vi "PID_controller_04.vi"() -> ()   [LabVIEW 2011]
uses:
  <vilib>/Platform/TimedLoop/XDataNode/nitl_modes.ctl
  <vilib>/Platform/TimedLoop/XDataNode/timing_clust.ctl
  <vilib>/Platform/TimedLoop/XDataNode/wakeup.ctl
  <vilib>/Platform/TimedLoop/XDataNode/XDataNode.xnode
  <vilib>/Platform/TimedLoop/XDataNode/XDNodeRunTimeDep.lvlib
panel:
  out "prev value":dbl
  out "Numeric":dbl
  out "x-y":dbl
  out "S00":dbl
  out "S10":dbl
  out "S20":dbl
  out "S11":dbl
  out "S01":dbl
  out "weight":dbl[](array[numeric])
  in  "# of points to watch":i32
  in  "alpha":dbl=-1.0
  out "t0":dbl
  out "error(t)":cluster{dbl, "Value":dbl}[](array[cluster])
  out "error out":errorcluster
  out "first":bool=TRUE
  out "P (torr)":string
  out "XY Graph":T1(graph)
  out "current value":dbl
  in  "stop":bool
  in  "Period (s)":dbl
  out "dValue":dbl
  out "derivative":dbl
  out "integral":dbl
  out "error":dbl
  out "Current angle (deg)":dbl
  in  "Kd":dbl
  in  "Ki":dbl
  in  "Kp":dbl
  out "Current P (torr)":dbl
  in  "Set Point (torr)":dbl
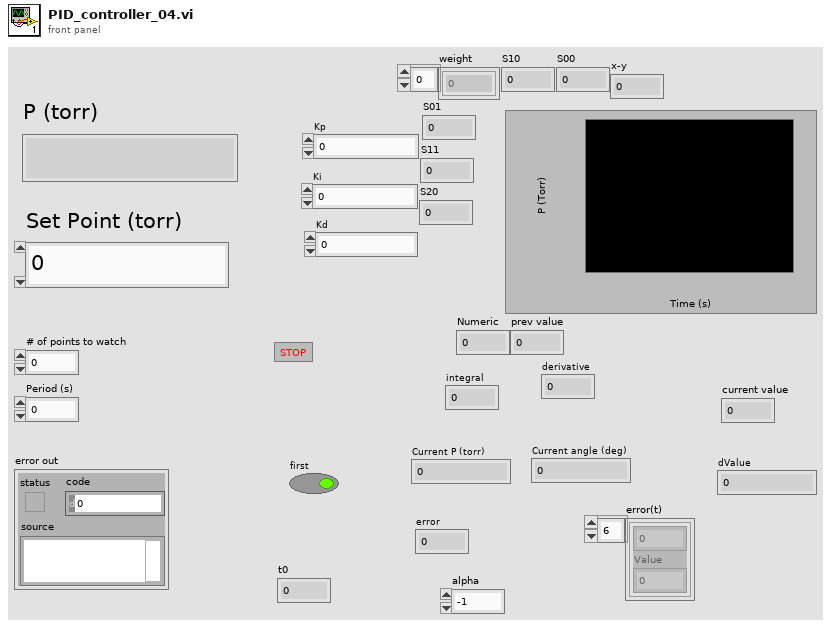
[diagram p1: front panel]
types:
  T1 = cluster{"Value":cluster{"element":dbl, "element":dbl}[]}[]
  T2 = typedef "XDNodeRunTimeDep.lvlib/nitl_modes.ctl" = enum32{"No Change", "Process missed periods, maintain original phase", "Discard missed periods, maintain original phase", "Process missed periods, ignore original phase", "Discard missed periods, ignore original phase"}
  T3 = typedef "XDNodeRunTimeDep.lvlib/timing_clust.ctl" = cluster{"Expected End [f-1]":u64, "Actual End [f-1]":u64, "Finished Late? [f-1]":bool, "Expected End [i-1]":u64, "Actual End [i-1]":u64, "Finished Late? [i-1]":bool, "Expected Start [i]":u64, "Actual Start [i]":u64, "Expected Start [f]":u64, "Actual Start [f]":u64, "Source Name":string, "Structure Name":string, "Period":i64, "Deadline":i64, "Offset":i64, "Start":i64, "Priority":i32, "Timeout":i32, "Mode":T2, "Wakeup Reason":T4, "Error":errorcluster, "Source Type":string, "Secondary Source Type":string, "Global End Time":u64, "Global Start Time":u64, "Frame Duration":u64, "Iteration Duration":u64, "Assigned CPU":i32, "I/O Scan Engine Mode":u32}
  T4 = typedef "XDNodeRunTimeDep.lvlib/wakeup.ctl" = enum32{"Normal", "Aborted", "Asynchronous wakeup", "Timing source error", "Timed loop error", "Timeout"}
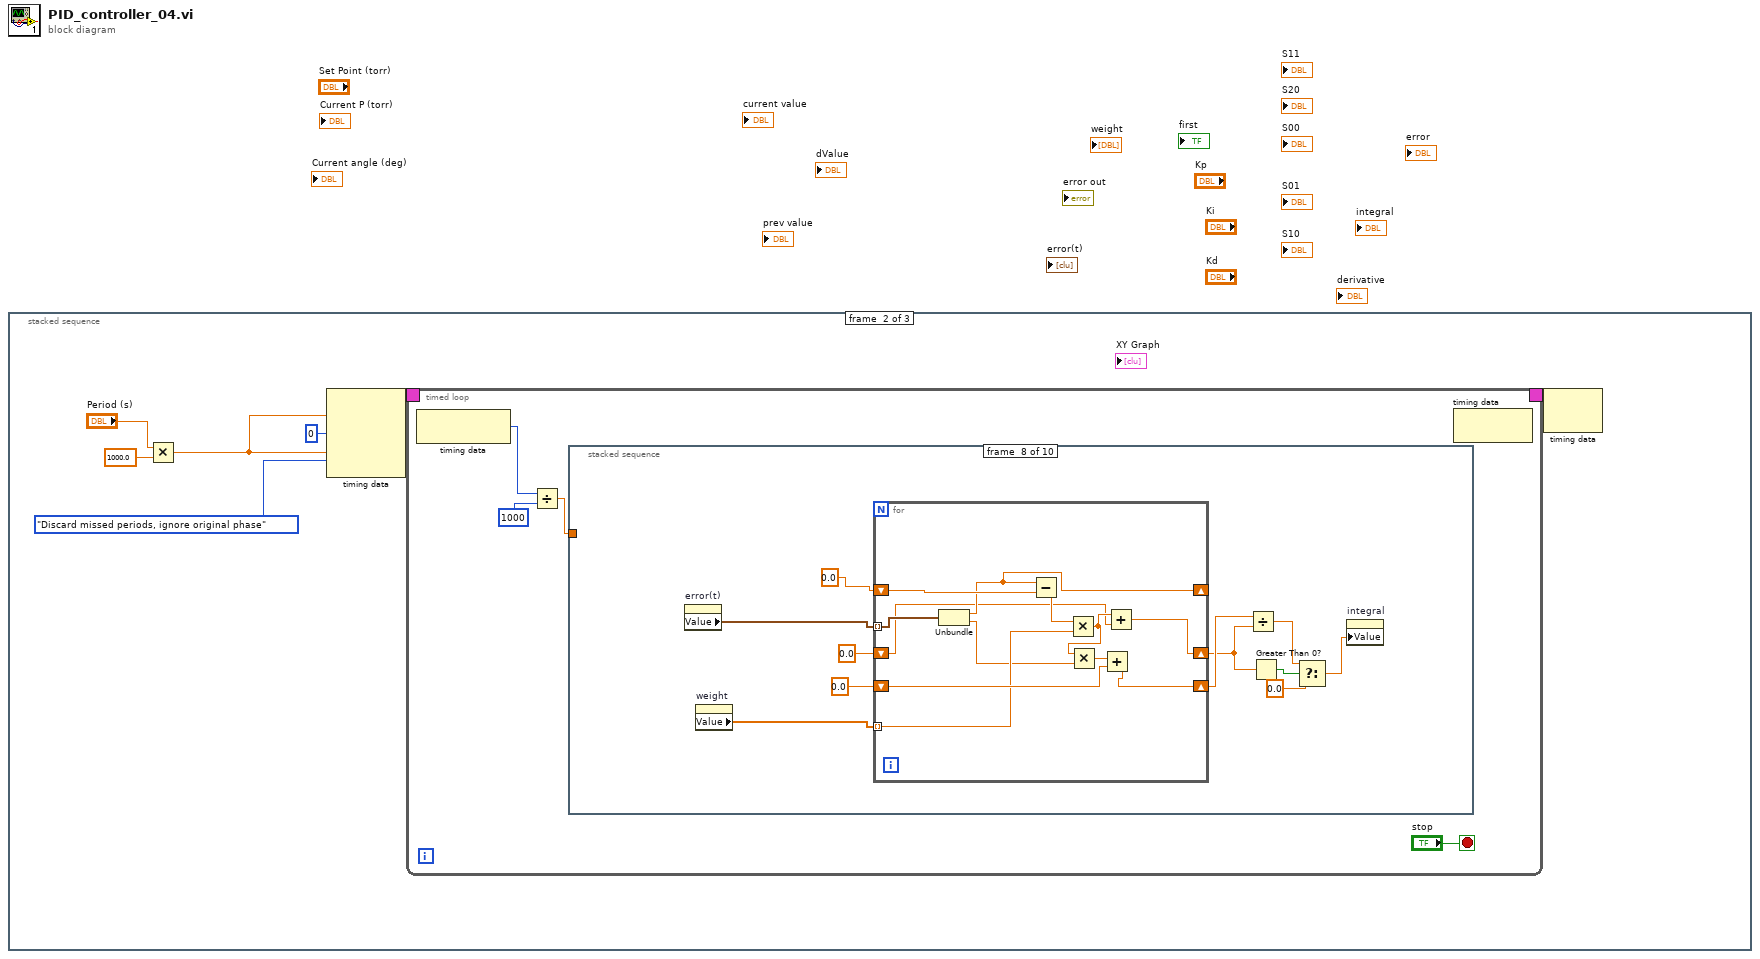
[diagram p0: block diagram]
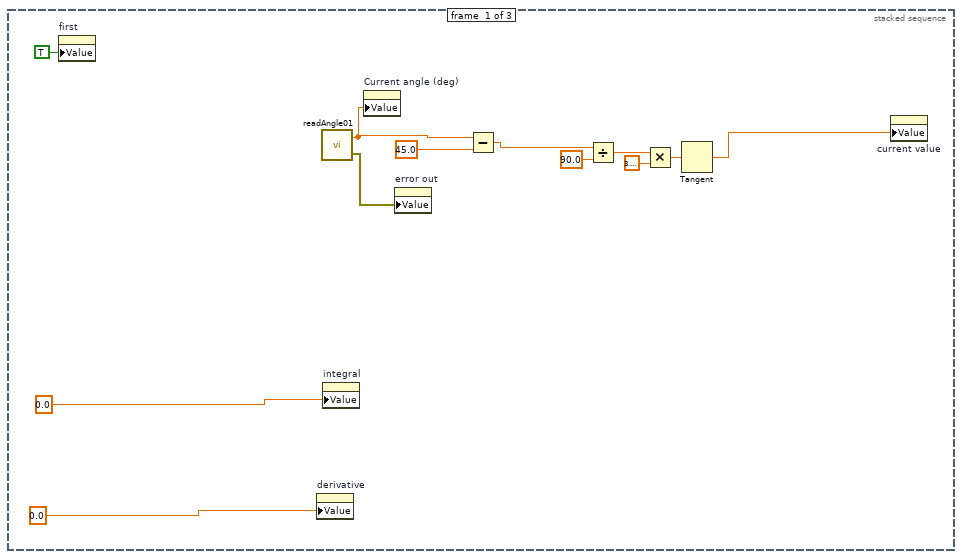
[diagram p2: hidden frame]
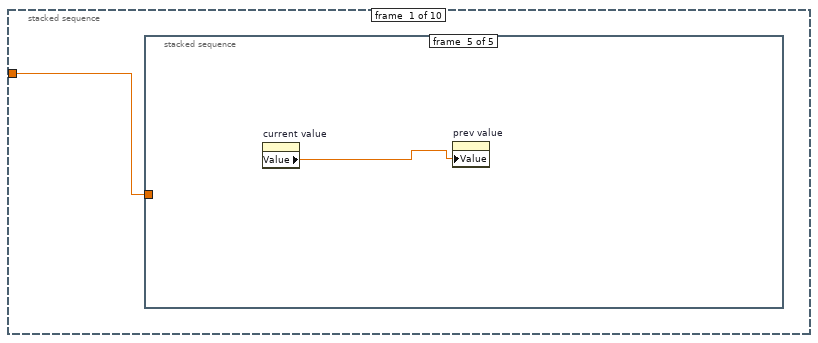
[diagram p3: hidden frame]
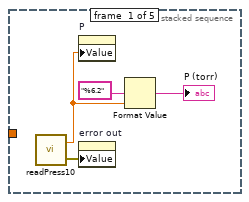
[diagram p4: hidden frame]
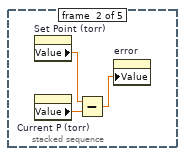
[diagram p5: hidden frame]
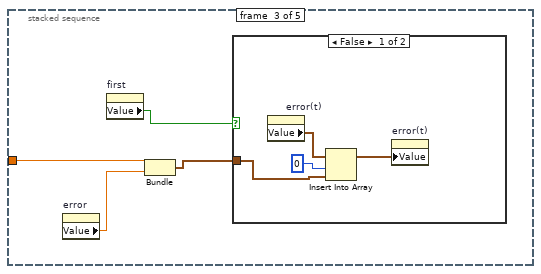
[diagram p6: hidden frame]
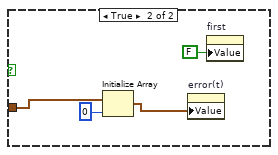
[diagram p7: hidden frame]
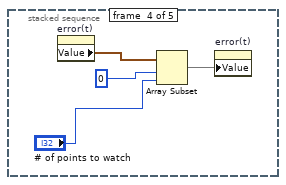
[diagram p8: hidden frame]
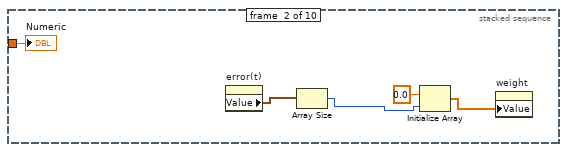
[diagram p9: hidden frame]
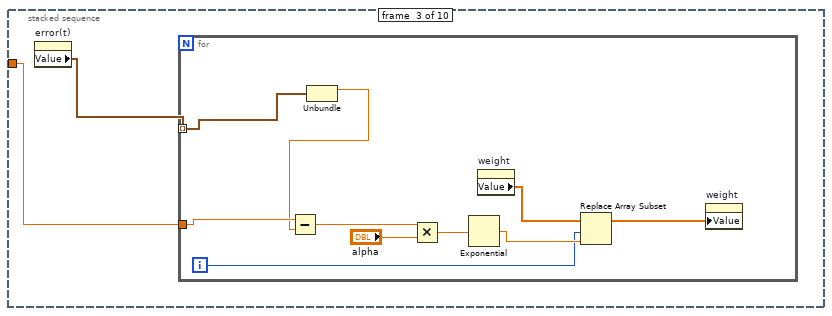
[diagram p10: hidden frame]
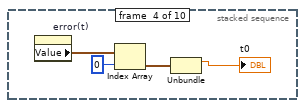
[diagram p11: hidden frame]
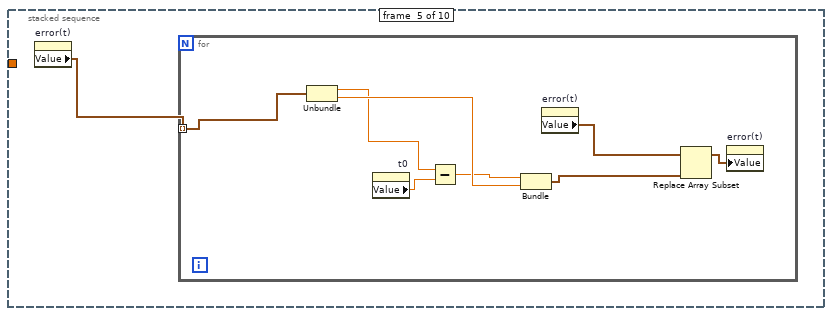
[diagram p12: hidden frame]
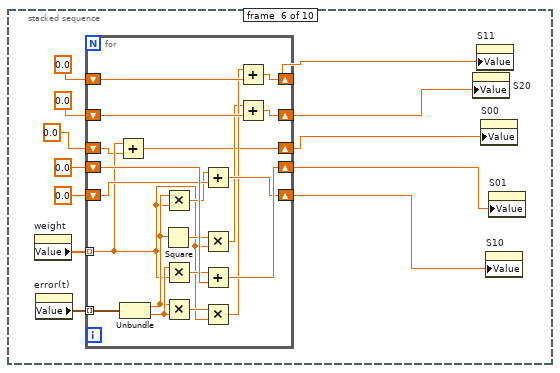
[diagram p13: hidden frame]
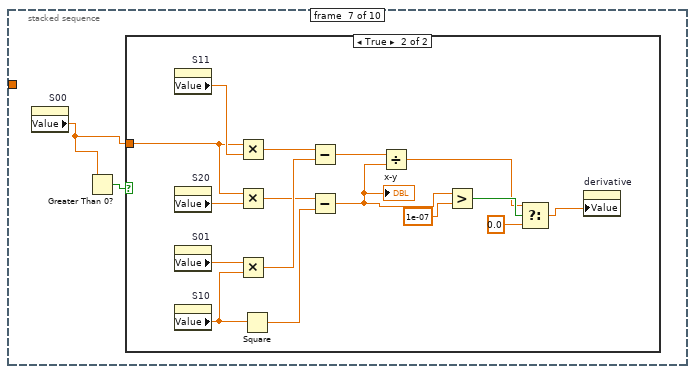
[diagram p14: hidden frame]
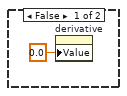
[diagram p15: hidden frame]
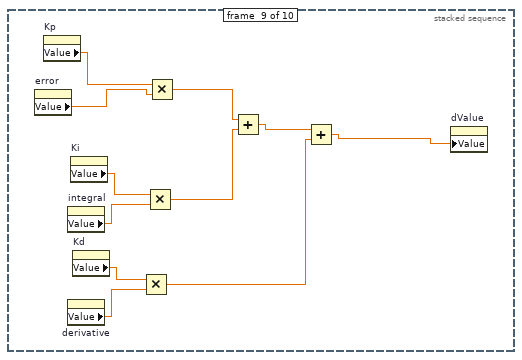
[diagram p16: hidden frame]
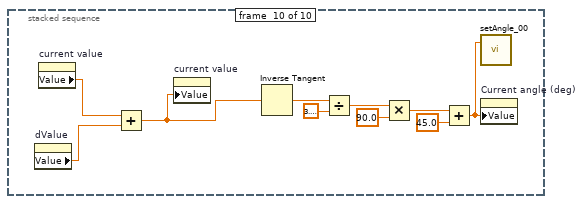
[diagram p17: hidden frame]
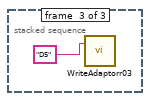
[diagram p18: hidden frame]
diagram:
  n1 = stacked-sequence {
    frame #0 {
      n2 = property on="first" class="Bool (strict)"("Value"=TRUE ("first")) -> ()  [unwired: 2 in, 2 out]
      n3 = property on="derivative" class="DigNum (strict)"("Value"=0.0 ("derivative")) -> ()  [unwired: 2 in, 2 out]
      n4 = call "readAngle01.vi"() -> ("angle"=w8:dbl, "error out"=w2:errorcluster)  [unwired: 1 in]
      n5 = property on="integral" class="DigNum (strict)"("Value"=0.0 ("integral")) -> ()  [unwired: 2 in, 2 out]
      n6 = property on="Current angle (deg)" class="DigNum (strict)"("Value"=w8) -> ()  [unwired: 2 in, 2 out]
      n7 = property on="error out" class="Clust (strict)"("Value"=w2) -> ()  [unwired: 2 in, 2 out]
      n8 = Subtract(x=w8, y=45.0) -> (x-y=w3:dbl)
      n9 = Divide(x=w3, y=90.0) -> (x/y=w6:dbl)
      n10 = Multiply(x=w6, y=3.141592653589793) -> (x*y=w4:dbl)
      n11 = Tangent(1:w4) -> (0:w1:dbl)
      n12 = property on="current value" class="DigNum (strict)"("Value"=w1) -> ()  [unwired: 2 in, 2 out]
    }
    frame #1 {
      n13 = Multiply(x="Period (s)", y=1000.0) -> (x*y=w14:dbl)
      n14 = node-c288(w14, i64 0 ("Offset"), w14, nitl_modes."Discard missed periods, ignore original phase" ("Mode")) -> (w19:T3)
      n15 = timed-loop {
        timing: w19 -> [_]
        timing-out: [_] -> w18
        stop <- "stop" stop-if-true
        n16 = node-c288() -> (w20:i64)  [unwired: 1 in]
        n17 = Divide(x=w20, y=i64 1000) -> (x/y=w21:dbl)
        n18 = stacked-sequence {
          tunnel: w21 -> [w24 w49 w54 _ _ _ _ _ _ _]
          frame #0 {
            n19 = stacked-sequence {
              tunnel: w24 -> [_ _ w34 _ _]
              frame #0 {
                n20 = call "readPress10.vi"() -> ("P"=w27:dbl, "error out"=w25:errorcluster)  [unwired: 1 in]
                n21 = property on="P" class="DigNum (strict)"("Value"=w27) -> ()  [unwired: 2 in, 2 out]
                n22 = property on="error out" class="Clust (strict)"("Value"=w25) -> ()  [unwired: 2 in, 2 out]
                n23 = Format Value(format string="%6.2", value (0)=w27) -> (output string=→"P (torr)":string)  [unwired: 1 in]
              }
              frame #1 {
                n24 = property on="Set Point (torr)" class="DigNum (strict)"() -> ("Value"=w30:dbl)  [unwired: 2 in, 2 out]
                n25 = property on="Current P (torr)" class="DigNum (strict)"() -> ("Value"=w31:dbl)  [unwired: 2 in, 2 out]
                n26 = Subtract(x=w30, y=w31) -> (x-y=w29:dbl)
                n27 = property on="error" class="DigNum (strict)"("Value"=w29) -> ()  [unwired: 2 in, 2 out]
              }
              frame #2 {
                n28 = property on="error" class="DigNum (strict)"() -> ("Value"=w33:dbl)  [unwired: 2 in, 2 out]
                n29 = property on="first" class="Bool (strict)"() -> ("Value"=w35:bool)  [unwired: 2 in, 2 out]
                n30 = Bundle(w34, "Value"=w33) -> (w32:cluster{dbl, "Value":dbl})  [unwired: 1 in]
                n31 = case shown="False" w35 {
                  tunnel: w32 -> [w36 w42]
                  frame False {
                    n32 = property on="error(t)" class="Arr (strict)"() -> ("Value"=w37:cluster{dbl, "Value":dbl}[])  [unwired: 2 in, 2 out]
                    n33 = Insert Into Array(array=w37, index=0, new element=w36) -> (w39:cluster{dbl, "Value":dbl}[])
                    n34 = property on="error(t)" class="Arr (strict)"("Value"=w39) -> ()  [unwired: 2 in, 2 out]
                  }
                  frame True {
                    n35 = Initialize Array(w42, 0 ("dimension size")) -> (w40:cluster{dbl, "Value":dbl}[])
                    n36 = property on="error(t)" class="Arr (strict)"("Value"=w40) -> ()  [unwired: 2 in, 2 out]
                    n37 = property on="first" class="Bool (strict)"("Value"=FALSE ("first")) -> ()  [unwired: 2 in, 2 out]
                  }
                }
              }
              frame #3 {
                n38 = property on="error(t)" class="Arr (strict)"() -> ("Value"=w45:cluster{dbl, "Value":dbl}[])  [unwired: 2 in, 2 out]
                n39 = Array Subset(array=w45, index=0, length="# of points to watch") -> (w47:cluster{dbl, "Value":dbl}[])
                n40 = property on="error(t)" class="Arr (strict)"("Value"=w47) -> ()  [unwired: 2 in, 2 out]
              }
              frame #4 {
                n41 = property on="current value" class="DigNum (strict)"() -> ("Value"=w48:dbl)  [unwired: 2 in, 2 out]
                n42 = property on="prev value" class="DigNum (strict)"("Value"=w48) -> ()  [unwired: 2 in, 2 out]
              }
            }
          }
          frame #1 {
            n43 = property on="error(t)" class="Arr (strict)"() -> ("Value"=w53:cluster{dbl, "Value":dbl}[])  [unwired: 2 in, 2 out]
            n44 = Array Size(array=w53) -> (size(s)=w51:i32)
            n45 = Initialize Array(0.0 ("element"), w51) -> (w50:dbl[])
            n46 = property on="weight" class="Arr (strict)"("Value"=w50) -> ()  [unwired: 2 in, 2 out]
            "Numeric" <- w49
          }
          frame #2 {
            n47 = property on="error(t)" class="Arr (strict)"() -> ("Value"=w55:cluster{dbl, "Value":dbl}[])  [unwired: 2 in, 2 out]
            n48 = for {
              tunnel: w55 -> [w65] mode=indexing
              tunnel: w54 -> [w62]
              i -> [w57]
              n49 = Unbundle(w65) -> (w61:dbl)  [unwired: 1 out]
              n50 = Subtract(x=w62, y=w61) -> (x-y=w60:dbl)
              n51 = Multiply(x=w60, y="alpha") -> (x*y=w63:dbl)
              n52 = Exponential(1:w63) -> (0:w59:dbl)
              n53 = property on="weight" class="Arr (strict)"() -> ("Value"=w58:dbl[])  [unwired: 2 in, 2 out]
              n54 = Replace Array Subset(array=w58, new element=w59, index=w57) -> (w56:dbl[])
              n55 = property on="weight" class="Arr (strict)"("Value"=w56) -> ()  [unwired: 2 in, 2 out]
            }
          }
          frame #3 {
            n56 = property on="error(t)" class="Arr (strict)"() -> ("Value"=w69:cluster{dbl, "Value":dbl}[])  [unwired: 2 in, 2 out]
            n57 = Index Array(array=w69, index=0) -> (element=w67:cluster{dbl, "Value":dbl})
            n58 = Unbundle(w67) -> (→"t0":dbl)  [unwired: 1 out]
          }
          frame #4 {
            n59 = property on="error(t)" class="Arr (strict)"() -> ("Value"=w70:cluster{dbl, "Value":dbl}[])  [unwired: 2 in, 2 out]
            n60 = for {
              tunnel: w70 -> [w75] mode=indexing
              n61 = Unbundle(w75) -> (w72:dbl, "Value"=w77:dbl)
              n62 = property on="t0" class="DigNum (strict)"() -> ("Value"=w78:dbl)  [unwired: 2 in, 2 out]
              n63 = Subtract(x=w72, y=w78) -> (x-y=w73:dbl)
              n64 = Bundle(w73, "Value"=w77) -> (w71:cluster{dbl, "Value":dbl})  [unwired: 1 in]
              n65 = property on="error(t)" class="Arr (strict)"() -> ("Value"=w76:cluster{dbl, "Value":dbl}[])  [unwired: 2 in, 2 out]
              n66 = Replace Array Subset(array=w76, new element=w71) -> (w74:cluster{dbl, "Value":dbl}[])  [unwired: 1 in]
              n67 = property on="error(t)" class="Arr (strict)"("Value"=w74) -> ()  [unwired: 2 in, 2 out]
            }
          }
          frame #5 {
            n68 = property on="weight" class="Arr (strict)"() -> ("Value"=w85:dbl[])  [unwired: 2 in, 2 out]
            n69 = property on="error(t)" class="Arr (strict)"() -> ("Value"=w90:cluster{dbl, "Value":dbl}[])  [unwired: 2 in, 2 out]
            n70 = for {
              tunnel: w90 -> [w106] mode=indexing
              shift-right: [w107] -> w80
              shift-left: 0.0 -> [w110]
              shift-right: [w103] -> w83
              shift-left: 0.0 -> [w109]
              shift-right: [w102] -> w82
              shift-left: 0.0 -> [w108]
              shift-right: [w104] -> w79
              shift-left: 0.0 -> [w105]
              tunnel: w85 -> [w93] mode=indexing
              shift-right: [w91] -> w81
              shift-left: 0.0 -> [w92]
              n71 = Add(x=w93, y=w92) -> (x+y=w91:dbl)
              n72 = Unbundle(w106) -> (w95:dbl, "Value"=w101:dbl)
              n73 = Square(x=w95) -> (x^2=w97:dbl)
              n74 = Multiply(x=w95, y=w93) -> (x*y=w94:dbl)
              n75 = Multiply(x=w101, y=w93) -> (x*y=w100:dbl)
              n76 = Multiply(x=w95, y=w101) -> (x*y=w99:dbl)
              n77 = Add(x=w94, y=w105) -> (x+y=w104:dbl)
              n78 = Multiply(x=w97, y=w93) -> (x*y=w96:dbl)
              n79 = Add(x=w100, y=w110) -> (x+y=w107:dbl)
              n80 = Multiply(x=w99, y=w93) -> (x*y=w98:dbl)
              n81 = Add(x=w98, y=w109) -> (x+y=w103:dbl)
              n82 = Add(x=w96, y=w108) -> (x+y=w102:dbl)
            }
            n83 = property on="S20" class="DigNum (strict)"("Value"=w82) -> ()  [unwired: 2 in, 2 out]
            n84 = property on="S11" class="DigNum (strict)"("Value"=w83) -> ()  [unwired: 2 in, 2 out]
            n85 = property on="S00" class="DigNum (strict)"("Value"=w81) -> ()  [unwired: 2 in, 2 out]
            n86 = property on="S10" class="DigNum (strict)"("Value"=w79) -> ()  [unwired: 2 in, 2 out]
            n87 = property on="S01" class="DigNum (strict)"("Value"=w80) -> ()  [unwired: 2 in, 2 out]
          }
          frame #6 {
            n88 = property on="S00" class="DigNum (strict)"() -> ("Value"=w111:dbl)  [unwired: 2 in, 2 out]
            n89 = Greater Than 0?(x=w111) -> (x > 0?=w112:bool)
            n90 = case shown="True" w112 {
              tunnel: w111 -> [_ w121]
              frame False {
                n91 = property on="derivative" class="DigNum (strict)"("Value"=0.0 ("derivative")) -> ()  [unwired: 2 in, 2 out]
              }
              frame True {
                n92 = property on="S11" class="DigNum (strict)"() -> ("Value"=w123:dbl)  [unwired: 2 in, 2 out]
                n93 = property on="S20" class="DigNum (strict)"() -> ("Value"=w122:dbl)  [unwired: 2 in, 2 out]
                n94 = property on="S01" class="DigNum (strict)"() -> ("Value"=w120:dbl)  [unwired: 2 in, 2 out]
                n95 = property on="S10" class="DigNum (strict)"() -> ("Value"=w124:dbl)  [unwired: 2 in, 2 out]
                n96 = Multiply(x=w121, y=w123) -> (x*y=w129:dbl)
                n97 = Multiply(x=w121, y=w122) -> (x*y=w127:dbl)
                n98 = Multiply(x=w120, y=w124) -> (x*y=w128:dbl)
                n99 = Square(x=w124) -> (x^2=w126:dbl)
                n100 = Subtract(x=w129, y=w128) -> (x-y=w125:dbl)
                n101 = Subtract(x=w127, y=w126) -> (x-y=w119:dbl)
                "x-y" <- w119
                n102 = Divide(x=w125, y=w119) -> (x/y=w115:dbl)
                n103 = Greater?(x=w119, y=1e-07) -> (0:w117:bool)
                n104 = Select(t=w115, s=w117, f=0.0) -> (s? t:f=w116:dbl)
                n105 = property on="derivative" class="DigNum (strict)"("Value"=w116) -> ()  [unwired: 2 in, 2 out]
              }
            }
          }
          frame #7 {
            n106 = property on="error(t)" class="Arr (strict)"() -> ("Value"=w140:cluster{dbl, "Value":dbl}[])  [unwired: 2 in, 2 out]
            n107 = property on="weight" class="Arr (strict)"() -> ("Value"=w138:dbl[])  [unwired: 2 in, 2 out]
            n108 = for {
              tunnel: w140 -> [w152] mode=indexing
              shift-right: [w150] -> _
              shift-left: 0.0 -> [w151]
              tunnel: w138 -> [w145] mode=indexing
              shift-right: [w146] -> w135
              shift-left: 0.0 -> [w147]
              shift-right: [w142] -> w134
              shift-left: 0.0 -> [w141]
              n109 = Unbundle(w152) -> (w150:dbl, "Value"=w144:dbl)
              n110 = Subtract(x=w150, y=w151) -> (x-y=w149:dbl)
              n111 = Multiply(x=w149, y=w145) -> (x*y=w143:dbl)
              n112 = Multiply(x=w143, y=w144) -> (x*y=w148:dbl)
              n113 = Add(x=w148, y=w147) -> (x+y=w146:dbl)
              n114 = Add(x=w143, y=w141) -> (x+y=w142:dbl)
            }
            n115 = Divide(x=w135, y=w134) -> (x/y=w132:dbl)
            n116 = Greater Than 0?(x=w134) -> (x > 0?=w133:bool)
            n117 = Select(t=w132, s=w133, f=0.0) -> (s? t:f=w130:dbl)
            n118 = property on="integral" class="DigNum (strict)"("Value"=w130) -> ()  [unwired: 2 in, 2 out]
          }
          frame #8 {
            n119 = property on="error" class="DigNum (strict)"() -> ("Value"=w163:dbl)  [unwired: 2 in, 2 out]
            n120 = property on="Kp" class="DigNum (strict)"() -> ("Value"=w162:dbl)  [unwired: 2 in, 2 out]
            n121 = property on="integral" class="DigNum (strict)"() -> ("Value"=w160:dbl)  [unwired: 2 in, 2 out]
            n122 = property on="derivative" class="DigNum (strict)"() -> ("Value"=w158:dbl)  [unwired: 2 in, 2 out]
            n123 = property on="Ki" class="DigNum (strict)"() -> ("Value"=w161:dbl)  [unwired: 2 in, 2 out]
            n124 = property on="Kd" class="DigNum (strict)"() -> ("Value"=w159:dbl)  [unwired: 2 in, 2 out]
            n125 = Multiply(x=w159, y=w158) -> (x*y=w155:dbl)
            n126 = Multiply(x=w161, y=w160) -> (x*y=w156:dbl)
            n127 = Multiply(x=w162, y=w163) -> (x*y=w157:dbl)
            n128 = Add(x=w157, y=w156) -> (x+y=w154:dbl)
            n129 = Add(x=w154, y=w155) -> (x+y=w153:dbl)
            n130 = property on="dValue" class="DigNum (strict)"("Value"=w153) -> ()  [unwired: 2 in, 2 out]
          }
          frame #9 {
            n131 = property on="dValue" class="DigNum (strict)"() -> ("Value"=w164:dbl)  [unwired: 2 in, 2 out]
            n132 = property on="current value" class="DigNum (strict)"() -> ("Value"=w165:dbl)  [unwired: 2 in, 2 out]
            n133 = Add(x=w165, y=w164) -> (x+y=w166:dbl)
            n134 = property on="current value" class="DigNum (strict)"("Value"=w166) -> ()  [unwired: 2 in, 2 out]
            n135 = Inverse Tangent(1:w166) -> (0:w173:dbl)
            n136 = Divide(x=w173, y=3.141592653589793) -> (x/y=w171:dbl)
            n137 = Multiply(x=w171, y=90.0) -> (x*y=w169:dbl)
            n138 = Add(x=w169, y=45.0) -> (x+y=w167:dbl)
            n139 = call "setAngle_00.vi"("Angle (deg)"=w167) -> ()  [unwired: 1 in, 1 out]
            n140 = property on="Current angle (deg)" class="DigNum (strict)"("Value"=w167) -> ()  [unwired: 2 in, 2 out]
          }
        }
        n141 = node-c288() -> ()  [unwired: 1 in, 1 out]
      }
      n142 = node-c288(w18) -> ()  [unwired: 1 out]
    }
    frame #2 {
      n143 = call "WriteAdaptorr03.vi"("string to write"="D5") -> ()  [unwired: 1 in, 1 out]
    }
  }
